vi "Enter.vi"(8 "error in (no error)":errorcluster, 11 "Wall":refnum<class "Wall.lvclass">) -> (0 "error out":errorcluster, 3 "Wall":refnum<class "Wall.lvclass">)   [LabVIEW 2020, in "Wall.lvclass"]
uses:
  Wall.lvclass
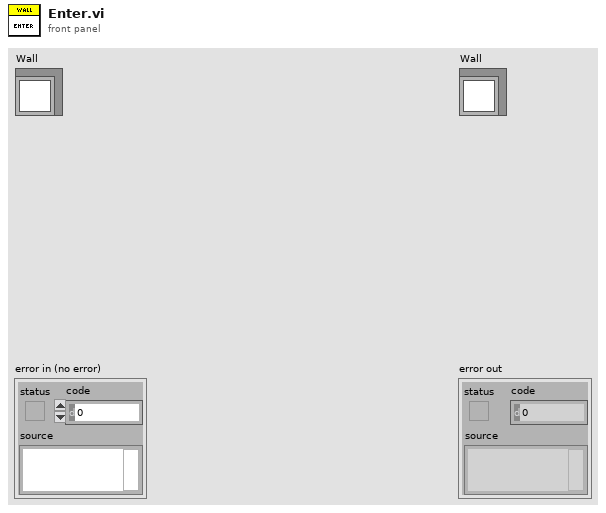
[diagram p1: front panel]
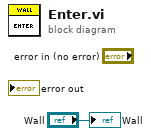
[diagram p0: block diagram]
diagram:
  "Wall" <- "Wall"
